vi "Controller Process.vi"(8 "error in (no error)":errorcluster, 10 "Queues":T1, 11 "UE Data Container":T2) -> (0 "error out":errorcluster)   [LabVIEW 2017]
doc: "Controller process of ATM."
uses:
  Shared Data/User Events/UE Data Container.ctl
  Error Handler/Controls/Error Data.ctl
  UIs/User Console/Controls/User Console - Transaction Enum.ctl
  Shared Data/Queues/Controls/Queues.ctl
  Controls/UI CMD.ctl
  Controls/Controller CMD.ctl
  Configuration/Controls/Config CMD.ctl
  Configuration/Controls/Config Data.ctl
  Controls/Controller Message Name.ctl
  UIs/Display Console/Controls/Display Data.ctl
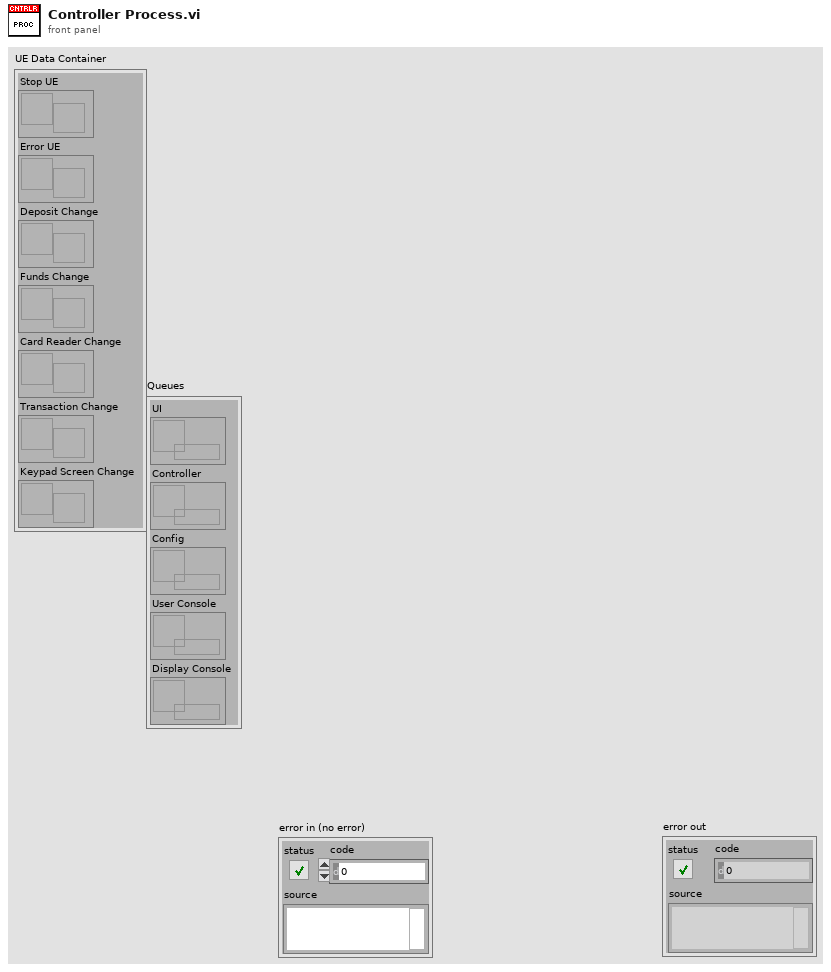
[diagram p1: front panel]
types:
  T1 = typedef "Queues.ctl" = cluster{"UI":refnum<queue>, "Controller":refnum<queue>, "Config":refnum<queue>, "User Console":refnum<queue>, "Display Console":refnum<queue>}
  T2 = typedef "UE Data Container.ctl" = cluster{"Stop UE":refnum<user-event>, "Error UE":refnum<user-event>, "Deposit Change":refnum<user-event>, "Funds Change":refnum<user-event>, "Card Reader Change":refnum<user-event>, "Transaction Change":refnum<user-event>, "Keypad Screen Change":refnum<user-event>}
  T3 = typedef "Config Data.ctl" = cluster{"Account Number":u32, "Last Name":string, "First Name":string, "Balance":dbl}
  T4 = cluster{"Messages":string[], "Config Data":T3, "Dynamic Data":string, "Invalid Login":i32}
  T5 = typedef "Controller CMD.ctl" = cluster{"Command":enum16{"Idle", "Init", "Config Update", "Terminate", "Send Message", "Login Start", "Login Finish", "Balance", "Deposit", "Withdrawal", "Fast Cash Start", "Fast Cash Stop", "Keypad Proc", "Search Account"}, "Data":variant}
  T6 = typedef "Controller Message Name.ctl" = enum16{"Welcome", "Login", "Idle", "Invalid Login", "Terminate", "Deposit", "Withdrawal", "Fast Cash", "Withdrawal Complete", "Withdrawal Failed", "Balance Inquiry"}
  T7 = typedef "Config CMD.ctl" = cluster{"CMD":enum16{"Idle", "Read", "Search", "Update", "Stop"}, "Data":variant}
  T8 = enum16{"Idle", "Init", "Config Update", "Terminate", "Send Message", "Login Start", "Login Finish", "Balance", "Deposit", "Withdrawal", "Fast Cash Start", "Fast Cash Stop", "Keypad Proc", "Search Account"}
  T9 = typedef "Display Data.ctl" = cluster{"Transaction":string, "Message":string, "Card Read":bool}
  T10 = enum16{"Idle", "Read", "Search", "Update", "Stop"}
  T11 = typedef "User Console - Transaction Enum.ctl" = enum16{"Balance Inquiry", "Deposit", "Withdrawal", "Fat Cash", "New Transaction", "Terminate Session"}
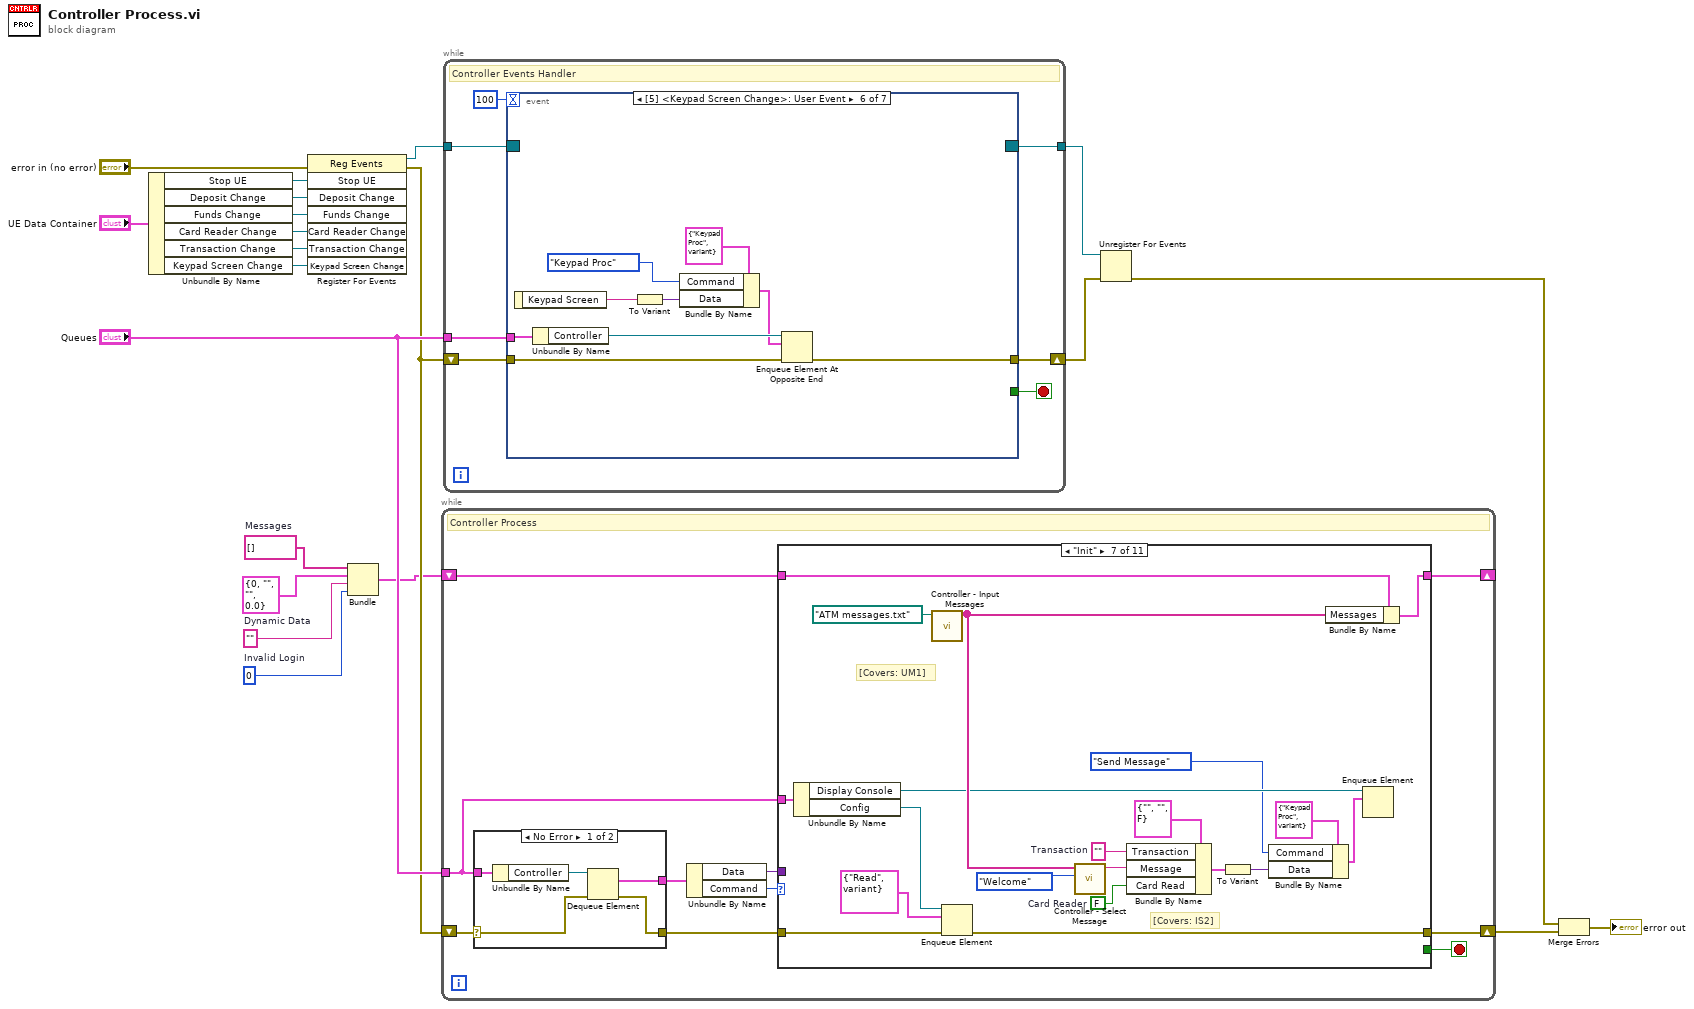
[diagram p0: block diagram]
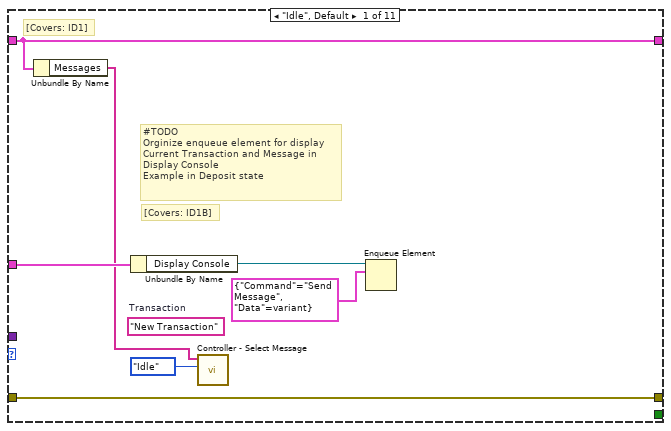
[diagram p2: hidden frame]
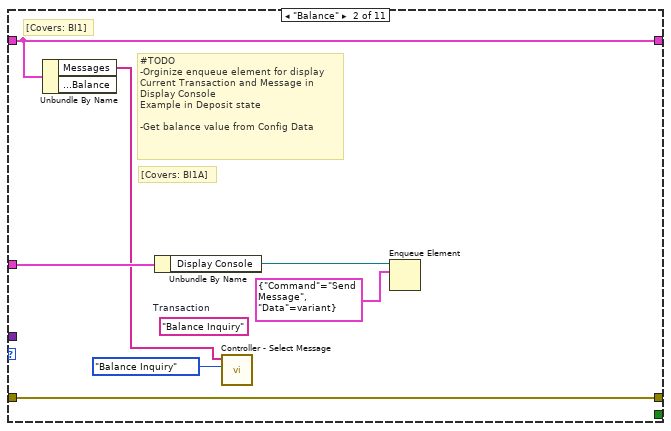
[diagram p3: hidden frame]
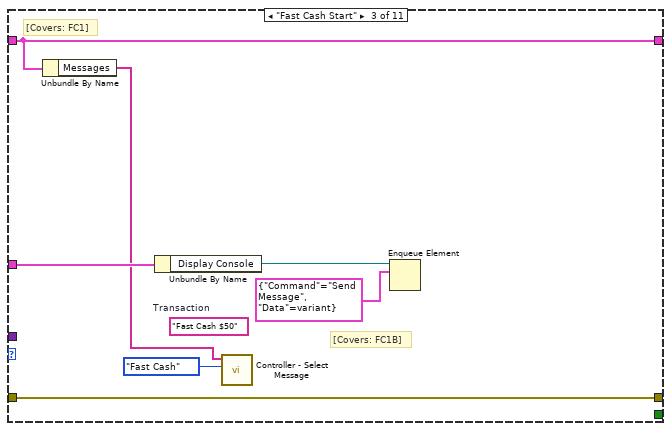
[diagram p4: hidden frame]
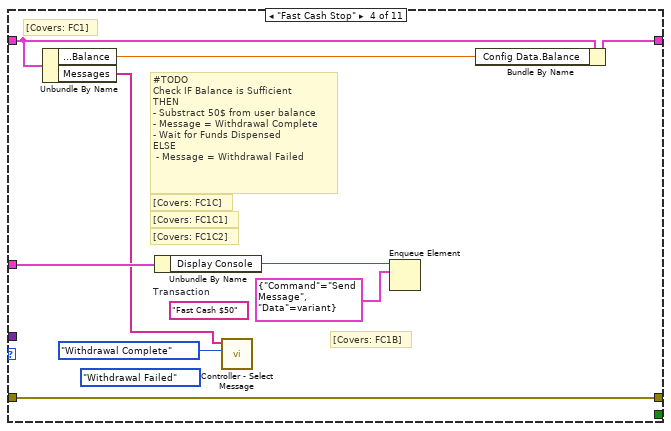
[diagram p5: hidden frame]
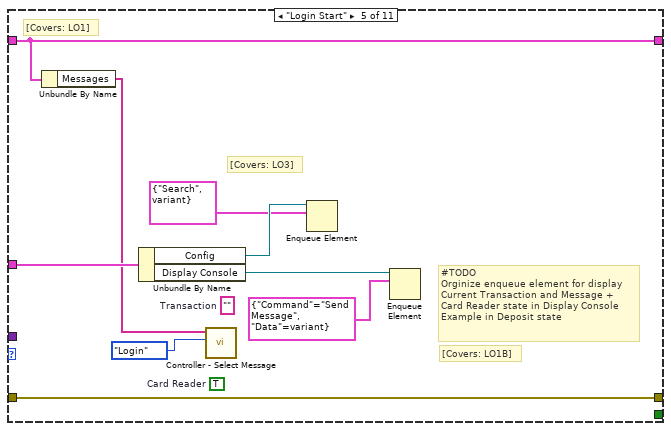
[diagram p6: hidden frame]
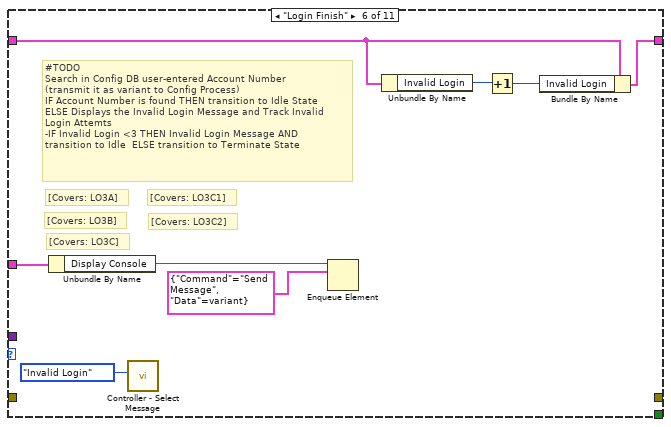
[diagram p7: hidden frame]
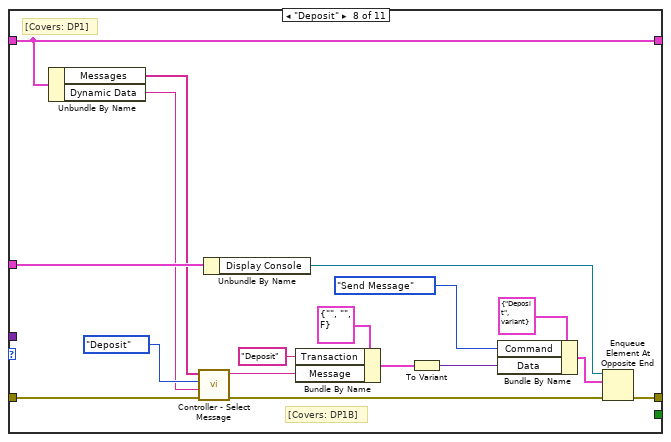
[diagram p8: hidden frame]
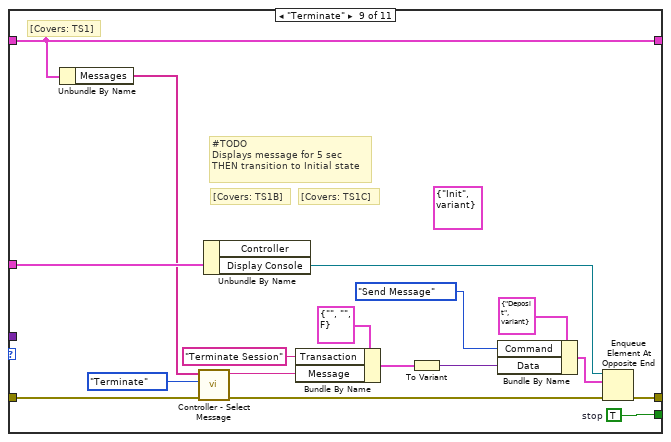
[diagram p9: hidden frame]
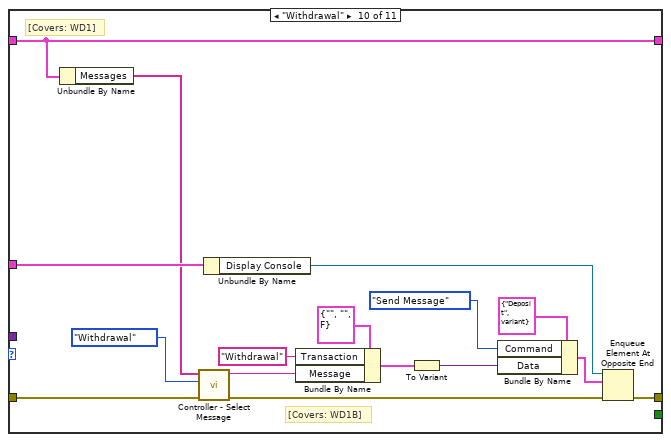
[diagram p10: hidden frame]
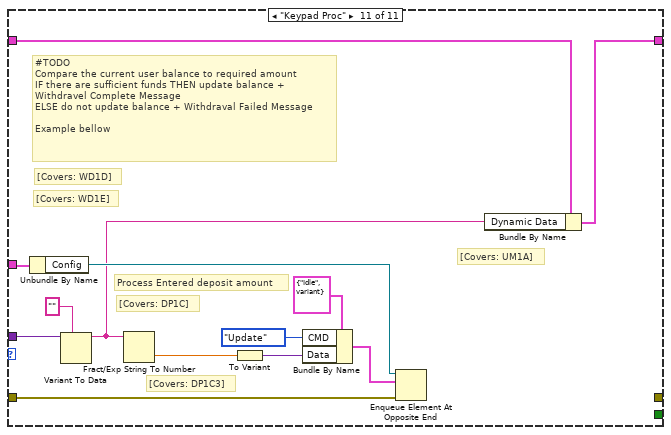
[diagram p11: hidden frame]
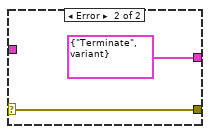
[diagram p12: hidden frame]
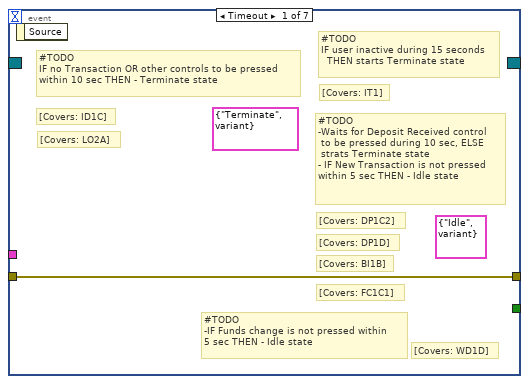
[diagram p13: hidden frame]
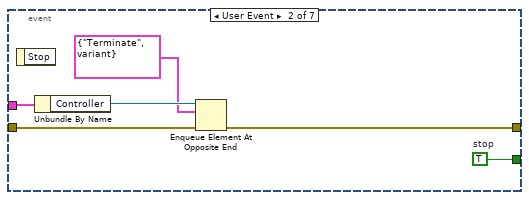
[diagram p14: hidden frame]
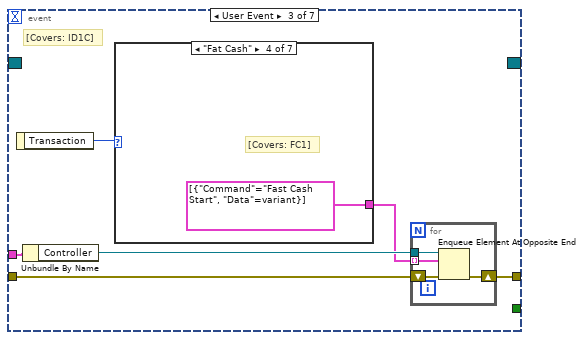
[diagram p15: hidden frame]
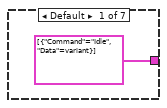
[diagram p16: hidden frame]
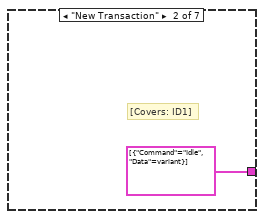
[diagram p17: hidden frame]
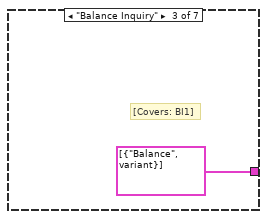
[diagram p18: hidden frame]
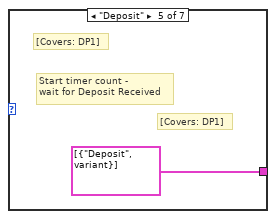
[diagram p19: hidden frame]
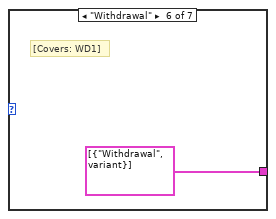
[diagram p20: hidden frame]
diagram:
  w1 = 0  # Invalid Login
  w2 = ""  # Dynamic Data
  w5 = string[] []  # Messages
  n1 = Unbundle By Name("UE Data Container") -> ("Stop UE"=w20:refnum<user-event>, "Deposit Change"=w6:refnum<user-event>, "Funds Change"=w7:refnum<user-event>, "Card Reader Change"=w8:refnum<user-event>, "Transaction Change"=w9:refnum<user-event>, "Keypad Screen Change"=w10:refnum<user-event>)
  n2 = register-events(error in="error in (no error)", w20, w6, w7, w8, w9, w10) -> (reference out=w18:refnum<event-registration>, error out=w14:errorcluster)  [unwired: 1 in]
  n3 = Bundle("Messages"=w5, "Config Data"=T3 {"Account Number"=0, "Last Name"="", "First Name"="", "Balance"=0.0}, "Dynamic Data"=w2, "Invalid Login"=w1) -> (w4:T4)  [unwired: 1 in]
  n4 = while {
    tunnel: "Queues" -> [w24]
    shift-right: [w26] -> w13
    shift-left: w14 -> [w31]
    shift-right: [w23] -> _
    shift-left: w4 -> [w22]
    stop <- w25 stop-if-true
    # "Controller Process"
    n5 = case shown="No Error" w31 {
      selector: w31 -> [w164 w168]
      tunnel: w24 -> [w166 _]
      tunnel: [w163 T5 {"Command"=enum."Terminate", "Data"=variant} ("Controller CMD")] -> w30
      tunnel: [w162 w168] -> w27
      frame No Error {
        n6 = Unbundle By Name(w166) -> ("Controller"=w165:refnum<queue>)
        n7 = Dequeue Element(queue=w165, error in (no error)=w164) -> (element=w163:T5, error out=w162:errorcluster)  [unwired: 1 in, 2 out]
      }
      frame Error {
      }
    }
    n8 = Unbundle By Name(w30) -> ("Data"=w28:variant, "Command"=w29:T8)
    n9 = case shown="\"Init\"" w29 {
      tunnel: w28 -> [_ _ _ _ _ _ _ _ _ _ w160]
      tunnel: w27 -> [w38 w45 w52 w61 w70 _ w94 w106 w123 w139 w158]
      tunnel: [w38 w45 w52 w61 w70 _ w93 w115 w132 w148 _] -> w26
      tunnel: [_ _ _ _ _ _ _ _ w117 _ _] -> w25
      tunnel: w24 -> [w36 w43 w50 w59 w68 w73 w95 w114 w131 w147 w157]
      tunnel: [w34 w41 w48 w54 w63 w75 w96 w102 w119 w135 w151] -> w23
      tunnel: w22 -> [w34 w41 w48 w57 w63 w76 w97 w102 w119 w135 w161]
      frame "Idle", Default {
        (unwired) "New Transaction"  # Transaction
        # "[Covers: ID1B]"
        # "#TODO\nOrginize enqueue element for display\nCurrent Transaction and Message in\nDisplay Console\nExample in Deposit state"
        # "[Covers: ID1]"
        n10 = Unbundle By Name(w34) -> ("Messages"=w33:string[])
        n11 = Unbundle By Name(w36) -> ("Display Console"=w35:refnum<queue>)
        n12 = call "Controller - Select Message.vi"("Message Name"=Controller_Message_Name."Idle", "Messages"=w33) -> ()  [unwired: 8 in, 2 out]
        n13 = Enqueue Element(queue=w35, element=T5 {"Command"=enum."Send Message", "Data"=variant}) -> ()  [unwired: 2 in, 3 out]
      }
      frame "Balance" {
        (unwired) "Balance Inquiry"  # Transaction
        # "[Covers: BI1A]"
        # "#TODO\n-Orginize enqueue element for display\nCurrent Transaction and Message in\nDisplay Console\nExample in Deposit state\n\n-Get balance value from Config Data"
        # "[Covers: BI1]"
        n14 = Unbundle By Name(w41) -> ("Messages"=w40:string[])  [unwired: 1 out]
        n15 = Unbundle By Name(w43) -> ("Display Console"=w42:refnum<queue>)
        n16 = call "Controller - Select Message.vi"("Message Name"=Controller_Message_Name."Balance Inquiry", "Messages"=w40) -> ()  [unwired: 8 in, 2 out]
        n17 = Enqueue Element(queue=w42, element=T5 {"Command"=enum."Send Message", "Data"=variant}) -> ()  [unwired: 2 in, 3 out]
      }
      frame "Fast Cash Start" {
        (unwired) "Fast Cash $50"  # Transaction
        # "[Covers: FC1B]"
        # "[Covers: FC1]"
        n18 = Unbundle By Name(w48) -> ("Messages"=w47:string[])
        n19 = Unbundle By Name(w50) -> ("Display Console"=w49:refnum<queue>)
        n20 = call "Controller - Select Message.vi"("Message Name"=Controller_Message_Name."Fast Cash", "Messages"=w47) -> ()  [unwired: 8 in, 2 out]
        n21 = Enqueue Element(queue=w49, element=T5 {"Command"=enum."Send Message", "Data"=variant}) -> ()  [unwired: 2 in, 3 out]
      }
      frame "Fast Cash Stop" {
        (unwired) Controller_Message_Name."Withdrawal Failed" ("Message Name")
        (unwired) "Fast Cash $50"  # Transaction
        # "[Covers: FC1C2]"
        # "[Covers: FC1C1]"
        # "[Covers: FC1C]"
        # "[Covers: FC1B]"
        # "#TODO\nCheck IF Balance is Sufficient \nTHEN\n- Substract 50$ from user balance\n- Message = Withdrawal Complete\n- Wait for Funds Dispensed\nELSE\n - Message = Withdrawal Failed"
        # "[Covers: FC1]"
        n22 = Unbundle By Name(w57) -> ("Config Data.Balance"=w53:dbl, "Messages"=w56:string[])
        n23 = Unbundle By Name(w59) -> ("Display Console"=w58:refnum<queue>)
        n24 = call "Controller - Select Message.vi"("Message Name"=Controller_Message_Name."Withdrawal Complete", "Messages"=w56) -> ()  [unwired: 8 in, 2 out]
        n25 = Enqueue Element(queue=w58, element=T5 {"Command"=enum."Send Message", "Data"=variant}) -> ()  [unwired: 2 in, 3 out]
        n26 = Bundle By Name(cluster=w57, "Config Data.Balance"=w53) -> (w54:T4)
      }
      frame "Login Start" {
        (unwired) TRUE  # Card Reader
        (unwired) ""  # Transaction
        # "[Covers: LO3]"
        # "[Covers: LO1B]"
        # "#TODO\nOrginize enqueue element for display\nCurrent Transaction and Message +\nCard Reader state in Display Console\nExample in Deposit state"
        # "[Covers: LO1]"
        n27 = Unbundle By Name(w63) -> ("Messages"=w62:string[])
        n28 = Unbundle By Name(w68) -> ("Config"=w66:refnum<queue>, "Display Console"=w67:refnum<queue>)
        n29 = call "Controller - Select Message.vi"("Message Name"=Controller_Message_Name."Login", "Messages"=w62) -> ()  [unwired: 8 in, 2 out]
        n30 = Enqueue Element(queue=w66, element=T7 {"CMD"=enum."Search", "Data"=variant}) -> ()  [unwired: 2 in, 3 out]
        n31 = Enqueue Element(queue=w67, element=T5 {"Command"=enum."Send Message", "Data"=variant}) -> ()  [unwired: 2 in, 3 out]
      }
      frame "Login Finish" {
        # "[Covers: LO3C2]"
        # "[Covers: LO3C1]"
        # "[Covers: LO3C]"
        # "[Covers: LO3B]"
        # "[Covers: LO3A]"
        # "#TODO\nSearch in Config DB user-entered Account Number\n(transmit it as variant to Config Process)\nIF Account Number is found THEN transition to Idle State\nELSE Displays the Invalid Login Message and Track Invalid \nLogin Attemts\n-IF Invalid Login <3 THEN Invalid Login Message AND \ntransition to Idle  ELSE transition to Terminate State"
        n32 = Unbundle By Name(w73) -> ("Display Console"=w72:refnum<queue>)
        n33 = call "Controller - Select Message.vi"("Message Name"=Controller_Message_Name."Invalid Login") -> ()  [unwired: 9 in, 2 out]
        n34 = Enqueue Element(queue=w72, element=T5 {"Command"=enum."Send Message", "Data"=variant}) -> ()  [unwired: 2 in, 3 out]
        n35 = Unbundle By Name(w76) -> ("Invalid Login"=w77:i32)
        n36 = Increment(x=w77) -> (x+1=w74:i32)
        n37 = Bundle By Name(cluster=w76, "Invalid Login"=w74) -> (w75:T4)
      }
      frame "Init" {
        w84 = FALSE  # Card Reader
        w86 = ""  # Transaction
        # "[Covers: IS2]"
        # "[Covers: UM1]"
        n38 = Unbundle By Name(w95) -> ("Display Console"=w88:refnum<queue>, "Config"=w92:refnum<queue>)
        n39 = call "Controller - Input Messages.vi"("FilePath"=path "ATM messages.txt") -> ("Messages"=w89:string[])  [unwired: 9 in, 1 out]
        n40 = Enqueue Element(queue=w92, element=T7 {"CMD"=enum."Read", "Data"=variant}, error in (no error)=w94) -> (error out=w93:errorcluster)  [unwired: 1 in, 2 out]
        n41 = call "Controller - Select Message.vi"("Message Name"=Controller_Message_Name."Welcome", "Messages"=w89) -> ("Message"=w85:string)  [unwired: 8 in, 1 out]
        n42 = Bundle By Name(cluster=T9 {"Transaction"="", "Message"="", "Card Read"=FALSE} ("Display Data"), "Transaction"=w86, "Message"=w85, "Card Read"=w84) -> (w83:T9)
        n43 = To Variant(anything=w83) -> (Variant=w82:variant)
        n44 = Bundle By Name(cluster=T5 {"Command"=enum."Keypad Proc", "Data"=variant} ("Controller CMD"), "Command"=T8."Send Message", "Data"=w82) -> (w80:T5)
        n45 = Bundle By Name(cluster=w97, "Messages"=w89) -> (w96:T4)
        n46 = Enqueue Element(queue=w88, element=w80) -> ()  [unwired: 2 in, 3 out]
      }
      frame "Deposit" {
        # "[Covers: DP1]"
        # "[Covers: DP1B]"
        n47 = Unbundle By Name(w102) -> ("Messages"=w101:string[], "Dynamic Data"=w100:string)
        n48 = call "Controller - Select Message.vi"("error in (no error)"=w106, "Dynamic Data"=w100, "Message Name"=Controller_Message_Name."Deposit", "Messages"=w101) -> ("error out"=w105:errorcluster, "Message"=w104:string)  [unwired: 6 in]
        n49 = Unbundle By Name(w114) -> ("Display Console"=w113:refnum<queue>)
        n50 = Bundle By Name(cluster=T9 {"Transaction"="", "Message"="", "Card Read"=FALSE} ("Display Data"), "Transaction"="Deposit", "Message"=w104) -> (w110:T9)
        n51 = To Variant(anything=w110) -> (Variant=w109:variant)
        n52 = Bundle By Name(cluster=T5 {"Command"=enum."Deposit", "Data"=variant} ("Controller CMD"), "Command"=T8."Send Message", "Data"=w109) -> (w108:T5)
        n53 = Enqueue Element At Opposite End(queue=w113, element=w108, error in (no error)=w105) -> (error out=w115:errorcluster)  [unwired: 1 in, 2 out]
      }
      frame "Terminate" {
        (unwired) T5 {"Command"=enum."Init", "Data"=variant} ("Controller CMD")
        w117 = TRUE  # stop
        # "[Covers: TS1C]"
        # "[Covers: TS1B]"
        # "#TODO\nDisplays message for 5 sec\nTHEN transition to Initial state"
        # "[Covers: TS1]"
        n54 = Unbundle By Name(w119) -> ("Messages"=w118:string[])
        n55 = call "Controller - Select Message.vi"("error in (no error)"=w123, "Message Name"=Controller_Message_Name."Terminate", "Messages"=w118) -> ("error out"=w122:errorcluster, "Message"=w121:string)  [unwired: 7 in]
        n56 = Unbundle By Name(w131) -> ("Display Console"=w130:refnum<queue>)  [unwired: 1 out]
        n57 = Bundle By Name(cluster=T9 {"Transaction"="", "Message"="", "Card Read"=FALSE} ("Display Data"), "Transaction"="Terminate Session", "Message"=w121) -> (w127:T9)
        n58 = To Variant(anything=w127) -> (Variant=w126:variant)
        n59 = Bundle By Name(cluster=T5 {"Command"=enum."Deposit", "Data"=variant} ("Controller CMD"), "Command"=T8."Send Message", "Data"=w126) -> (w125:T5)
        n60 = Enqueue Element At Opposite End(queue=w130, element=w125, error in (no error)=w122) -> (error out=w132:errorcluster)  [unwired: 1 in, 2 out]
      }
      frame "Withdrawal" {
        # "[Covers: WD1]"
        # "[Covers: WD1B]"
        n61 = Unbundle By Name(w135) -> ("Messages"=w134:string[])
        n62 = call "Controller - Select Message.vi"("error in (no error)"=w139, "Message Name"=Controller_Message_Name."Withdrawal", "Messages"=w134) -> ("error out"=w138:errorcluster, "Message"=w137:string)  [unwired: 7 in]
        n63 = Unbundle By Name(w147) -> ("Display Console"=w146:refnum<queue>)
        n64 = Bundle By Name(cluster=T9 {"Transaction"="", "Message"="", "Card Read"=FALSE} ("Display Data"), "Transaction"="Withdrawal", "Message"=w137) -> (w143:T9)
        n65 = To Variant(anything=w143) -> (Variant=w142:variant)
        n66 = Bundle By Name(cluster=T5 {"Command"=enum."Deposit", "Data"=variant} ("Controller CMD"), "Command"=T8."Send Message", "Data"=w142) -> (w141:T5)
        n67 = Enqueue Element At Opposite End(queue=w146, element=w141, error in (no error)=w138) -> (error out=w148:errorcluster)  [unwired: 1 in, 2 out]
      }
      frame "Keypad Proc" {
        # "[Covers: UM1A]"
        # "[Covers: WD1E]"
        # "[Covers: WD1D]"
        # "#TODO\nCompare the current user balance to required amount\nIF there are sufficient funds THEN update balance + \nWithdravel Complete Message\nELSE do not update balance + Withdraval Failed Message\n\nExample bellow"
        # "[Covers: DP1C]"
        # "Process Entered deposit amount"
        # "[Covers: DP1C3]"
        n68 = Unbundle By Name(w157) -> ("Config"=w156:refnum<queue>)
        n69 = Variant To Data(type="", Variant=w160) -> (data=w149:string)  [unwired: 1 in, 1 out]
        n70 = Fract/Exp String To Number(string=w149) -> (number=w150:dbl)  [unwired: 3 in, 1 out]
        n71 = To Variant(anything=w150) -> (Variant=w155:variant)
        n72 = Bundle By Name(cluster=T7 {"CMD"=enum."Idle", "Data"=variant} ("Config CMD"), "CMD"=T10."Update", "Data"=w155) -> (w152:T7)
        n73 = Enqueue Element At Opposite End(queue=w156, element=w152, error in (no error)=w158) -> ()  [unwired: 1 in, 3 out]
        n74 = Bundle By Name(cluster=w161, "Dynamic Data"=w149) -> (w151:T4)
      }
    }
  }
  n75 = while {
    tunnel: w18 -> [w175]
    tunnel: [w174] -> w17
    tunnel: "Queues" -> [w172]
    shift-right: [w170] -> w16
    shift-left: w14 -> [w171]
    stop <- w173 stop-if-true
    # "Controller Events Handler"
    n76 = event shown="[5] <Keypad Screen Change>: User Event" {
      selector: w175 -> [_ _ _ _ _ _ _]
      dyn-events: [_ _ _ _ _ _ _] -> w174
      timeout: 100 -> [_ _ _ _ _ _ _]
      tunnel: [_ w182 _ _ _ _ _] -> w173
      tunnel: w172 -> [_ w181 w187 _ w205 w214 w219]
      tunnel: w171 -> [w176 w179 w186 w200 w203 w212 w218]
      tunnel: [w176 w178 w184 w200 w202 w211 w217] -> w170
      event Timeout {
        (unwired) T5 {"Command"=enum."Terminate", "Data"=variant} ("Controller CMD")
        (unwired) T5 {"Command"=enum."Idle", "Data"=variant} ("Controller CMD")
        # "[Covers: FC1C1]"
        # "[Covers: BI1B]"
        # "[Covers: LO2A]"
        # "[Covers: ID1C]"
        # "#TODO\nIF no Transaction OR other controls to be pressed\nwithin 10 sec THEN - Terminate state"
        # "[Covers: WD1D]"
        # "#TODO\n-IF Funds change is not pressed within\n5 sec THEN - Idle state"
        # "[Covers: DP1D]"
        # "[Covers: DP1C2]"
        # "#TODO\n-Waits for Deposit Received control\n to be pressed during 10 sec, ELSE\n strats Terminate state\n- IF New Transaction is not pressed\nwithin 5 sec THEN - Idle state"
        # "[Covers: IT1]"
        # "#TODO\nIF user inactive during 15 seconds\n  THEN starts Terminate state"
        n77 = event-data() -> ()  [unwired: 1 in, 1 out]
      }
      event User Event {
        w182 = TRUE  # stop
        n78 = event-data() -> ()  [unwired: 1 in, 1 out]
        n79 = Unbundle By Name(w181) -> ("Controller"=w180:refnum<queue>)
        n80 = Enqueue Element At Opposite End(queue=w180, element=T5 {"Command"=enum."Terminate", "Data"=variant} ("Controller CMD"), error in (no error)=w179) -> (error out=w178:errorcluster)  [unwired: 1 in, 2 out]
      }
      event User Event {
        # "[Covers: ID1C]"
        n81 = event-data() -> ("Transaction"=w188:T11)  [unwired: 1 in]
        n82 = Unbundle By Name(w187) -> ("Controller"=w185:refnum<queue>)
        n83 = case shown="\"Fat Cash\"" w188 {
          tunnel: [T5[] [{"Command"=enum."Idle", "Data"=variant}] T5[] [{"Command"=enum."Idle", "Data"=variant}] T5[] [{"Command"=enum."Balance", "Data"=variant}] T5[] [{"Command"=enum."Fast Cash Start", "Data"=variant}] T5[] [{"Command"=enum."Deposit", "Data"=variant}] T5[] [{"Command"=enum."Withdrawal", "Data"=variant}] T5[] [{"Command"=enum."Terminate", "Data"=variant}]] -> w183
          frame Default {
          }
          frame "New Transaction" {
            # "[Covers: ID1]"
          }
          frame "Balance Inquiry" {
            # "[Covers: BI1]"
          }
          frame "Fat Cash" {
            # "[Covers: FC1]"
          }
          frame "Deposit" {
            # "[Covers: DP1]"
            # "[Covers: DP1]"
            # "Start timer count - \nwait for Deposit Received"
          }
          frame "Withdrawal" {
            # "[Covers: WD1]"
          }
          frame "Terminate Session" {
            # "[Covers: TS1]"
          }
        }
        n84 = for {
          tunnel: w185 -> [w191]
          tunnel: w183 -> [w189] mode=indexing
          shift-right: [w190] -> w184
          shift-left: w186 -> [w192]
          n85 = Enqueue Element At Opposite End(queue=w191, element=w189, error in (no error)=w192) -> (error out=w190:errorcluster)  [unwired: 1 in, 2 out]
        }
      }
      event User Event {
        n86 = event-data() -> ()  [unwired: 1 in, 1 out]
      }
      event User Event {
        # "[Covers: WD1D]"
        # "Wait for the User event and return to Idle state"
        n87 = event-data() -> ()  [unwired: 1 in, 1 out]
        n88 = Unbundle By Name(w205) -> ("Controller"=w204:refnum<queue>)
        n89 = Enqueue Element At Opposite End(queue=w204, element=T5 {"Command"=enum."Idle", "Data"=variant} ("Controller CMD"), error in (no error)=w203) -> (error out=w202:errorcluster)  [unwired: 1 in, 2 out]
      }
      event User Event {
        n90 = event-data() -> ("Keypad Screen"=w209:string)  [unwired: 1 in]
        n91 = Unbundle By Name(w214) -> ("Controller"=w213:refnum<queue>)
        n92 = To Variant(anything=w209) -> (Variant=w207:variant)
        n93 = Bundle By Name(cluster=T5 {"Command"=enum."Keypad Proc", "Data"=variant} ("Controller CMD"), "Command"=T8."Keypad Proc", "Data"=w207) -> (w208:T5)
        n94 = Enqueue Element At Opposite End(queue=w213, element=w208, error in (no error)=w212) -> (error out=w211:errorcluster)  [unwired: 1 in, 2 out]
      }
      event User Event {
        # "[Covers: LO1]"
        n95 = event-data() -> ()  [unwired: 1 in, 1 out]
        n96 = Unbundle By Name(w219) -> ("Controller"=w216:refnum<queue>)
        n97 = for {
          tunnel: w216 -> [w222]
          tunnel: T5[] [{"Command"=enum."Login Start", "Data"=variant}] -> [w220] mode=indexing
          shift-right: [w221] -> w217
          shift-left: w218 -> [w223]
          n98 = Enqueue Element At Opposite End(queue=w222, element=w220, error in (no error)=w223) -> (error out=w221:errorcluster)  [unwired: 1 in, 2 out]
        }
      }
    }
  }
  n99 = Unregister For Events(event registration refnum=w17, error in=w16) -> (error out=w12:errorcluster)
  n100 = Merge Errors(w12, w13) -> (→"error out":errorcluster)
